vi "NextState.vi"(8 "Error In":errorcluster, 9 "Data":variant, 10 "State":string, 11 "Queue In":refnum<queue>) -> (0 "Error Out":errorcluster, 3 "Queue Out":refnum<queue>)   [LabVIEW 2016]
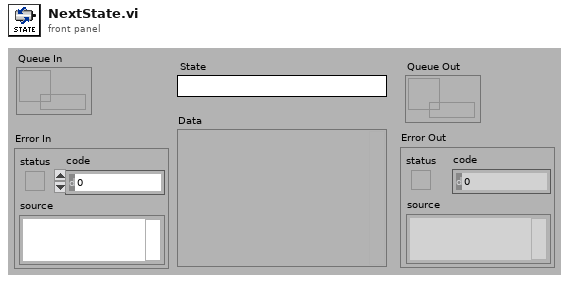
[diagram p1: front panel]
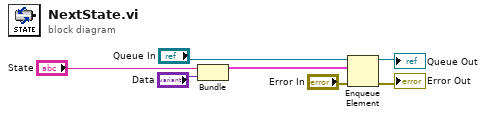
[diagram p0: block diagram]
diagram:
  n1 = Bundle("State"="State", "Data"="Data") -> (w5:cluster{"State":string, "Data":variant})  [unwired: 1 in]
  n2 = Enqueue Element(queue="Queue In", element=w5, error in (no error)="Error In") -> (queue out=→"Queue Out":refnum<queue>, error out=→"Error Out":errorcluster)  [unwired: 1 in, 1 out]
